vi "G#Object_ConvertFlattenedDataToMoreGeneric.vi"(0 "reference in":refnum<class "G#Object.lvclass">, 1 "full class name":string, 3 "type string":i16[](array[numeric]), 5 "error in (no error)":errorcluster) -> (14 "reference converterrd":refnum<class "G#Object.lvclass">, 19 "error out":errorcluster)   [LabVIEW 2020, in "G#Object.lvclass"]
doc: "Converts the reference in to the more generic class specifiec by the full class name."
uses:
  G#Object.lvclass
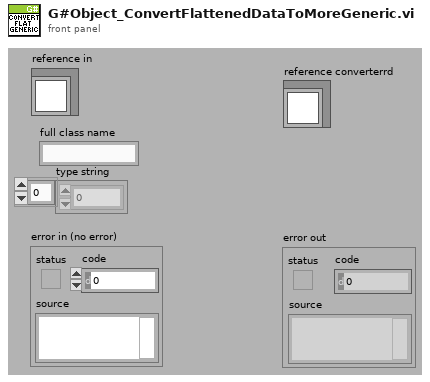
[diagram p1: front panel]
types:
  T1 = typedef "G#Object.lvclass/G#Object_ClassHierarchy.ctl" = cluster{"ClassName":string, "FullClassName":string, "ClassPath":path, "IsLeaf":bool}
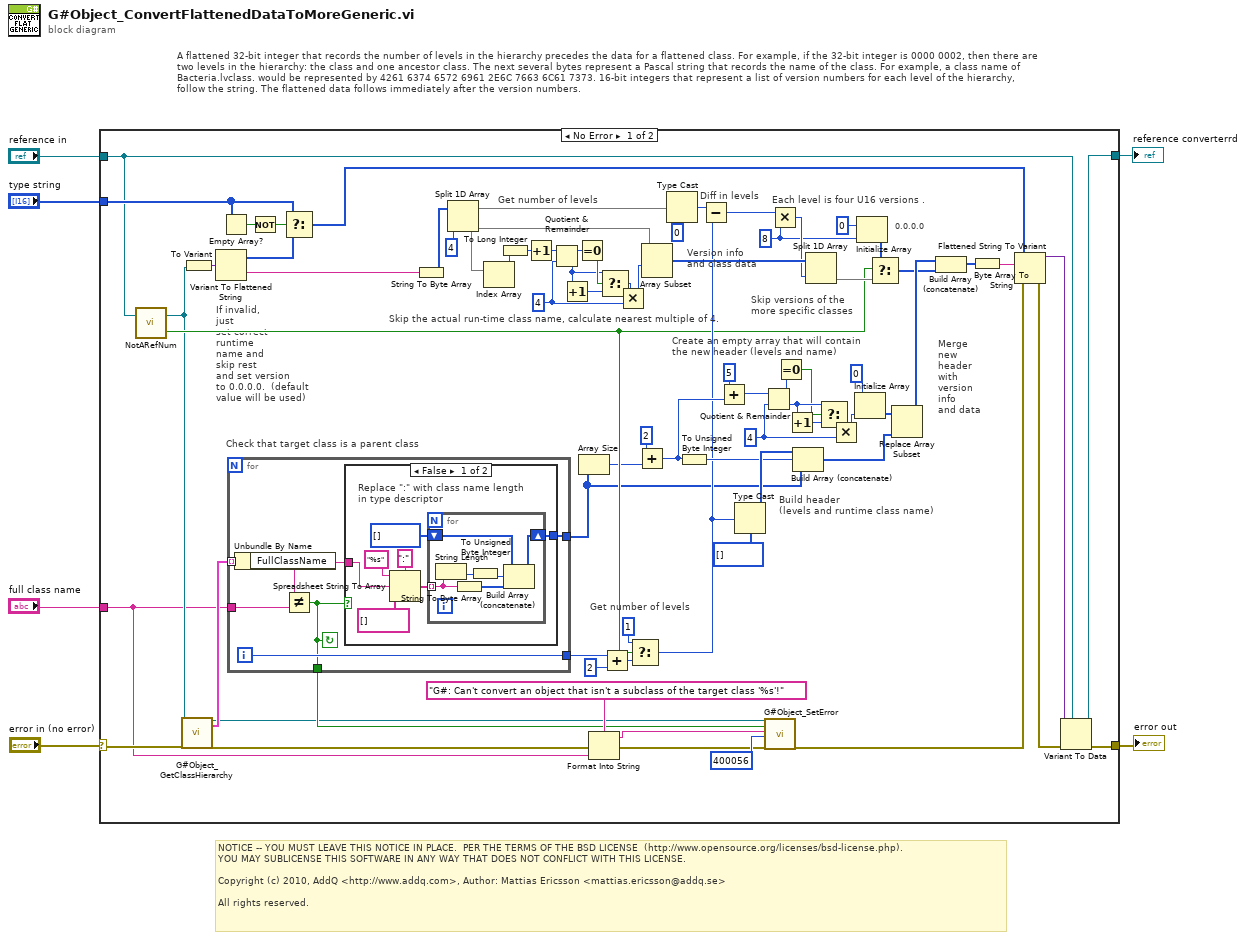
[diagram p0: block diagram]
diagram:
  # "A flattened 32-bit integer that records the number of levels in the hierarchy precedes the data for a flattened class. For example, if the 32-bit integer is 0000 0002, then there are two levels in the hierarchy: the class and one ancestor class. The next several bytes represent a Pascal string that records the name of the class. For example, a class name of Bacteria.lvclass. would be represented by 4261 6374 6572 6961 2E6C 7663 6C61 7373. 16-bit integers that represent a list of version numbers for each level of the hierarchy, follow the string. The flattened data follows immediately after the version numbers."
  # "NOTICE -- YOU MUST LEAVE THIS NOTICE IN PLACE.  PER THE TERMS OF THE BSD LICENSE  (http://www.opensource.org/licenses/bsd-license.php).\nYOU MAY SUBLICENSE THIS SOFTWARE IN ANY WAY THAT DOES NOT CONFLICT WITH THIS LICENSE.\n\nCopyright (c) 2010, AddQ <http://www.addq.com>, Author: Mattias Ericsson <mattias.ericsson@addq.se>\n\nAll rights reserved."
  n1 = case shown="No Error" "error in (no error)" {
    selector: "error in (no error)" -> [w28 w103]
    tunnel: [w20 w103] -> w4
    tunnel: "full class name" -> [w7 _]
    tunnel: "reference in" -> [w18 w102]
    tunnel: "type string" -> [w23 _]
    tunnel: [w17 w102] -> w1
    frame No Error {
      w46 = 4 ("y")
      w33 = 8 ("y")
      w49 = 4 ("y")
      # "0.0.0.0"
      # "If invalid,\njust\nset correct\nruntime\nname and\nskip rest\nand set version\nto 0.0.0.0.  (default\nvalue will be used)"
      # "Each level is four U16 versions ."
      # "Merge\nnew\nheader\nwith\nversion\ninfo\nand data"
      # "Build header\n(levels and runtime class name)"
      # "Create an empty array that will contain\nthe new header (levels and name)"
      # "Skip versions of the\nmore specific classes"
      # "Diff in levels"
      # "Get number of levels"
      # "Version info\nand class data"
      # "Skip the actual run-time class name, calculate nearest multiple of 4."
      # "Get number of levels"
      # "Check that target class is a parent class"
      n2 = call-dynamic "NotARefNum.vi"("reference in"=w18) -> ("not a refnum?"=w34:bool, "reference out"=w10:refnum<class "G#Object.lvclass">)  [unwired: 1 in]
      n3 = call "G#Object_GetClassHierarchy.vi"("reference in"=w10, "error in (no error)"=w28) -> ("reference out"=w9:refnum<class "G#Object.lvclass">, "class hierarchy"=w82:T1[], "error out"=w12:errorcluster)  [unwired: 15 in]
      n4 = To Variant(anything=w10) -> (Variant=w81:variant)
      n5 = Variant To Flattened String(Variant=w81) -> (data string=w45:string, 1:w24:i16[])
      n6 = Empty Array?(array=w23) -> (empty?=w26:bool)
      n7 = for {
        tunnel: w82 -> [w88] mode=indexing
        tunnel: w7 -> [w85]
        tunnel: [w87] -> w80
        tunnel: [w86] -> w11
        tunnel: [w83] -> w30
        i -> [w87]
        stop <- w86 continue-if-true
        n8 = Unbundle By Name(w88) -> ("FullClassName"=w84:string)
        n9 = Not Equal?(x=w84, y=w85) -> (x != y?=w86:bool)
        n10 = case shown="False" w86 {
          tunnel: w84 -> [w93 _]
          tunnel: [w89 _] -> w83
          frame False {
            # "Replace \":\" with class name length\nin type descriptor"
            n11 = Spreadsheet String To Array(delimiter (Tab)=":", format string="%s", spreadsheet string=w93, array type (2D Dbl)=string[] []) -> (array=w91:string[])
            n12 = for {
              tunnel: w91 -> [w100] mode=indexing
              shift-right: [w97] -> w89
              shift-left: u8[] [] -> [w96]
              n13 = String Length(string=w100) -> (length=w101:i32)
              n14 = String To Byte Array(string=w100) -> (unsigned byte array=w98:u8[])
              n15 = To Unsigned Byte Integer(number=w101) -> (unsigned 8bit integer=w99:u8)
              n16 = Build Array (concatenate)(w96, w99, w98) -> (w97:u8[])
            }
          }
          frame True {
          }
        }
      }
      n17 = Not(x=w26) -> (.not. x?=w25:bool)
      n18 = Select(t=w23, s=w25, f=w24) -> (s? t:f=w22:i16[])
      n19 = String To Byte Array(string=w45) -> (unsigned byte array=w69:u8[])
      n20 = Split 1D Array(array=w69, index=4 ("length")) -> (first subarray=w71:u8[], second subarray=w42:u8[])
      n21 = Index Array(array=w42) -> (element=w78:u8)  [unwired: 1 in]
      n22 = To Long Integer(number=w78) -> (32bit integer=w41:i32)
      n23 = Increment(x=w41) -> (x+1=w40:i32)
      n24 = Quotient & Remainder(x=w40, y=w49) -> (x-y*floor(x/y)=w77:i32, floor(x/y)=w74:i32)
      n25 = Increment(x=w74) -> (x+1=w75:i32)
      n26 = Equal To 0?(x=w77) -> (x = 0?=w76:bool)
      n27 = Array Size(array=w30) -> (size(s)=w29:i32)
      n28 = Format Into String(format string="G#: Can't convert an object that isn't a subclass of the target class '%s'!", error in=w12, w7) -> (resulting string=w13:string, error out=w14:errorcluster)  [unwired: 1 in]
      n29 = Select(t=w74, s=w76, f=w75) -> (s? t:f=w51:i32)
      n30 = Add(x=w80, y=2) -> (x+y=w39:i32)
      n31 = Multiply(x=w51, y=w49) -> (x*y=w50:i32)
      n32 = Select(t=1, s=w34, f=w39) -> (s? t:f=w38:i32)
      n33 = Add(x=2, y=w29) -> (x+y=w58:i32)
      n34 = Array Subset(array=w42, index=w50) -> (w66:u8[])  [unwired: 1 in]
      n35 = Type Cast(type=0 ("y"), x=w71) -> (*(type *) &x=w68:i32)
      n36 = To Unsigned Byte Integer(number=w58) -> (unsigned 8bit integer=w57:u8)
      n37 = Subtract(x=w68, y=w38) -> (x-y=w67:i32)
      n38 = Add(x=5, y=w58) -> (x+y=w60:i32)
      n39 = Type Cast(type=u8[] [] ("unsigned byte array"), x=w38) -> (*(type *) &x=w59:u8[])
      n40 = Quotient & Remainder(x=w60, y=w46) -> (x-y*floor(x/y)=w61:i32, floor(x/y)=w64:i32)
      n41 = call "G#Object_SetError.vi"("reference in"=w9, "error (F)"=w11, "source"=w13, "code"=400056, "error in (no error)"=w14) -> ("error out"=w8:errorcluster)  [unwired: 14 in]
      n42 = Multiply(x=w67, y=w33) -> (x*y=w44:i32)
      n43 = Equal To 0?(x=w61) -> (x = 0?=w62:bool)
      n44 = Increment(x=w64) -> (x+1=w63:i32)
      n45 = Build Array (concatenate)(w59, w57, w30) -> (w54:u8[])
      n46 = Split 1D Array(array=w66, index=w44) -> (second subarray=w36:u8[])  [unwired: 1 out]
      n47 = Select(t=w64, s=w62, f=w63) -> (s? t:f=w48:i32)
      n48 = Multiply(x=w48, y=w46) -> (x*y=w47:i32)
      n49 = Initialize Array(u8 0, w47) -> (w55:u8[])
      n50 = Initialize Array(u8 0, w33) -> (w32:u8[])
      n51 = Select(t=w32, s=w34, f=w36) -> (s? t:f=w35:u8[])
      n52 = Replace Array Subset(array=w55, new element=w54) -> (w53:u8[])  [unwired: 1 in]
      n53 = Build Array (concatenate)(w53, w35) -> (w52:u8[])
      n54 = Byte Array To String(unsigned byte array=w52) -> (string=w27:string)
      n55 = Flattened String To Variant(4:w8, 6:w27, 7:w22) -> (0:w21:errorcluster, 3:w19:variant)
      n56 = Variant To Data(error in=w21, type=w18, Variant=w19) -> (data=w17:refnum<class "G#Object.lvclass">, error out=w20:errorcluster)
    }
    frame Error {
    }
  }
  "error out" <- w4
  "reference converterrd" <- w1
